vi "Complex To Polar - RM.vi"(0 "Real Matrix r*e^i0":T1) -> (1 "Modulus r":T1, 2 "Argument Q (0)":T1)   [LabVIEW 2017, in "NI_Matrix.lvlib"]
doc: "Breaks a complex number into its polar components."
uses:
  NI_Matrix.lvlib
  RealMatrix.ctl
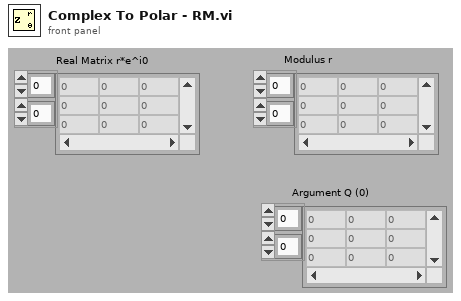
[diagram p1: front panel]
types:
  T1 = typedef "NI_Matrix.lvlib/RealMatrix.ctl" = dbl[][]
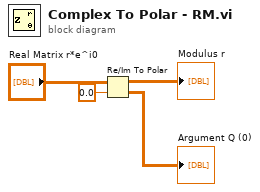
[diagram p0: block diagram]
diagram:
  n1 = Re/Im To Polar(2:0.0 ("element"), 3:"Real Matrix r*e^i0") -> (0:→"Argument Q (0)":T1, 1:→"Modulus r":T1)
